vi "Remove All Ports.vi"(8 "error in":errorcluster, 11 "custom device ref":T1 format="%.0x") -> (0 "error out":errorcluster, 3 "custom device ref out":T1 format="%.0x")   [LabVIEW 2020, in "Ballard ARINC 429 Scripting.lvlib"]
uses:
  Ballard ARINC 429 Scripting.lvlib
  <vilib>/NI VeriStand/Custom Device API/Custom Device Item Ref.ctl
  <vilib>/NI VeriStand/Custom Device API/Custom Device API.lvlib
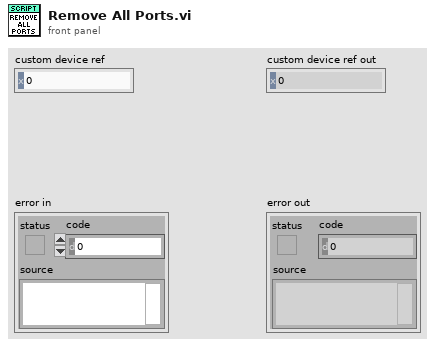
[diagram p1: front panel]
types:
  T1 = typedef "Custom Device API.lvlib/Custom Device Item Ref.ctl" = u64
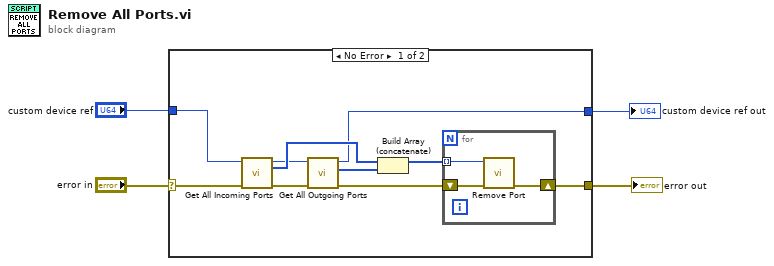
[diagram p0: block diagram]
diagram:
  n1 = case shown="No Error" "error in" {
    selector: "error in" -> [w14 w19]
    tunnel: [w10 w19] -> w4
    tunnel: "custom device ref" -> [w13 w18]
    tunnel: [w6 w18] -> w1
    frame No Error {
      n2 = call "Get All Incoming Ports.vi"("error in"=w14, "Ballard ARINC 429 ref"=w13) -> ("error out"=w12:errorcluster, "Port refs"=w8:T1[], "Ballard ARINC 429 ref out"=w7:T1)  [unwired: 7 in]
      n3 = call "Get All Outgoing Ports.vi"("error in"=w12, "Ballard ARINC 429 ref"=w7) -> ("error out"=w11:errorcluster, "Port refs"=w9:T1[], "Ballard ARINC 429 ref out"=w6:T1)  [unwired: 7 in]
      n4 = Build Array (concatenate)(w8, w9) -> (w5:T1[])
      n5 = for {
        shift-right: [w16] -> w10
        shift-left: w11 -> [w17]
        tunnel: w5 -> [w15] mode=indexing
        n6 = call "Remove Port.vi"("error in"=w17, "port ref"=w15) -> ("error out"=w16:errorcluster)  [unwired: 9 in]
      }
    }
    frame Error {
    }
  }
  "error out" <- w4
  "custom device ref out" <- w1
